vi "Output_StepMotor.vi"() -> ()   [LabVIEW 2018]
uses:
  <vilib>/DAQmx/create/channels.llb/DAQmx Create Channel (CO-Pulse Generation-Frequency).vi
  <vilib>/DAQmx/configure/timing.llb/DAQmx Timing (Implicit).vi
panel:
  in  "정지":bool
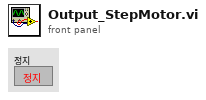
[diagram p1: front panel]
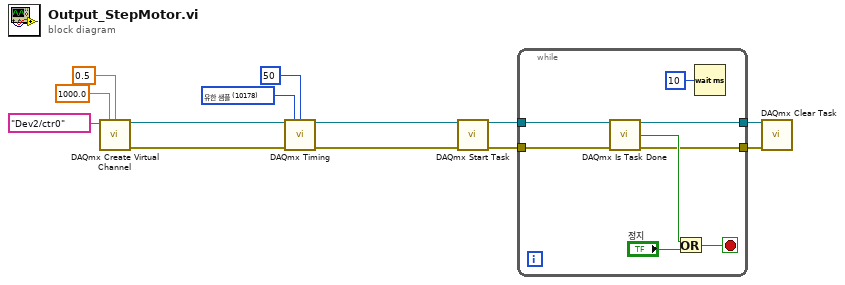
[diagram p0: block diagram]
diagram:
  w3 = 10178 items=["유한 샘플"=10178, "연속 샘플"=10123, "하드웨어 타이밍에 의한 단일 포인트"=12522] ("sample mode")
  n1 = call-poly <vilib>:"DAQmx Create Virtual Channel.vi"("frequency"=1000.0, "duty cycle"=0.5, "counter"=tag "Dev2/ctr0") -> ("task out"=w13:refnum<k21>, "error out"=w12:errorcluster)  [unwired: 11 in]
  n2 = call-poly <vilib>:"DAQmx Timing.vi"("task/channels in"=w13, "sample mode"=w3, "samples per channel"=50, "error in"=w12) -> ("task out"=w11:refnum<k21>, "error out"=w10:errorcluster)  [unwired: 10 in]
  n3 = call <vilib>:"DAQmx Start Task.vi"("task/channels in"=w11, "error in"=w10) -> ("task out"=w9:refnum<k21>, "error out"=w8:errorcluster)  [unwired: 12 in]
  n4 = while {
    tunnel: w9 -> [w18]
    tunnel: w8 -> [w17]
    tunnel: [w16] -> w7
    tunnel: [w15] -> w6
    stop <- w20 stop-if-true
    n5 = call <vilib>:"DAQmx Is Task Done.vi"("task/channels in"=w18, "error in"=w17) -> ("task out"=w16:refnum<k21>, "task done?"=w19:bool, "error out"=w15:errorcluster)  [unwired: 11 in]
    n6 = Or(x=w19, y="정지") -> (x .or. y?=w20:bool)
    n7 = Wait (ms)(milliseconds to wait=u32 10 ("대기 시간 (ms)")) -> ()  [unwired: 1 out]
  }
  n8 = call <vilib>:"DAQmx Clear Task.vi"("task in"=w7, "error in"=w6) -> ()  [unwired: 13 in, 1 out]
